vi "channel.set_metadata.vi"(4 "clear_unit":bool, 5 "data_type":i32, 6 "unit":string, 7 "data source rid":string, 8 "error in":errorcluster, 9 "description":string, 10 "name":string, 11 "Client in":refnum<class "Client.lvclass">) -> (0 "error out":errorcluster, 2 "Channel":refnum<class "Channel.lvclass">, 3 "Client out":refnum<class "Client.lvclass">)   [LabVIEW 2020, in "Client.lvclass"]
doc: "Sets a channel's data type, description, and unit, creating the metadata record if it doesn't already exist."
uses:
  Client.lvclass
  Client.lvclass/Client.ctl
  client.lvlib
  Channel/Channel.lvclass
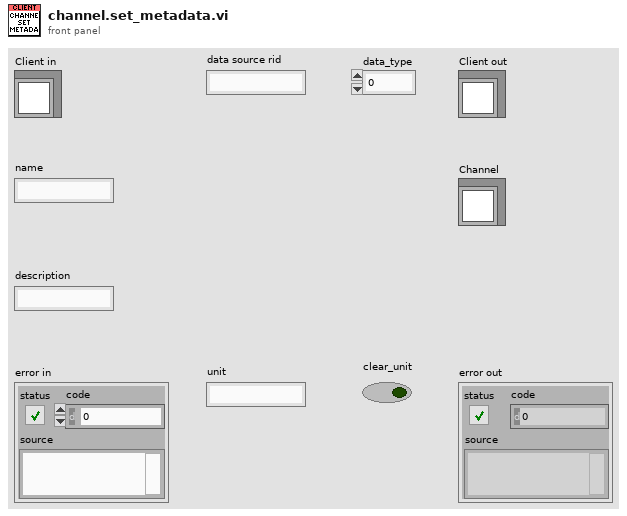
[diagram p1: front panel]
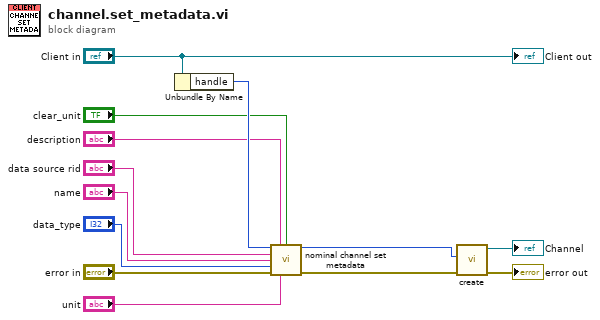
[diagram p0: block diagram]
diagram:
  n1 = Unbundle By Name("Client in") -> ("handle"=w12:i32)
  n2 = call "nominal channel set metadata.vi"("client"=w12, "description"="description", "clear_unit"="clear_unit", "data_source_rid"="data source rid", "name"="name", "data_type"="data_type", "error in (no error)"="error in", "unit"="unit") -> ("out_channel out"=w4:i32, "error out"=w1:errorcluster)  [unwired: 5 in, 1 out]
  n3 = call "create.vi"("error in (no error)"=w1, "handle"=w4) -> ("error out"=→"error out":errorcluster, "Channel"=→"Channel":refnum<class "Channel.lvclass">)  [unwired: 8 in]
  "Client out" <- "Client in"
